vi "LVAPT_Git_Item_OnPopupMenu.vi"(11 "Object":T1) -> ()   [LabVIEW 2019]
uses:
  <resource>/Framework/Providers/API/ItemRef.ctl
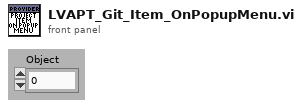
[diagram p1: front panel]
types:
  T1 = typedef "ItemRef.ctl" = u64
  T2 = enum32{"<None>", "Project", "Project / Build Specifications", "Tools", "Tools / Source Control", "Tools / Real-Time Module", "Help"}
  T3 = typedef "mxLvMenuItem.ctl" = cluster{"Menu Name":string, "Description":string, "Icon File Name":path, "Menu Tag":string, "Enabled":bool, "Checked":bool, "Separator":bool, "Batchable":bool, "Weight":i32, "Batch Mode (Ignored if Not Batchable)":enum32{"Show If All Items Support Command", "Show If Any Items Support Command"}, "Menu Location":enum32{"<None>", "Project", "Project / Build Specifications", "Tools", "Tools / Source Control", "Tools / Real-Time Module", "Help"}, "Exclude From Getting Started Window Menu":bool}
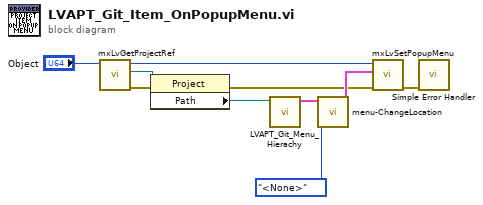
[diagram p0: block diagram]
diagram:
  n1 = call <resource>:"mxLvGetProjectRef.vi"("Item"="Object") -> ("error out"=w6:errorcluster, "Project Refnum"=w5:refnum<vi>, "Item"=w4:T1)  [unwired: 8 in]
  n2 = property class="Project"(reference=w5, error in=w6) -> (error out=w1:errorcluster, "Path"=w2:path)  [unwired: 1 out]
  n3 = call "LVAPT_Git_Menu_Hierachy.vi"("ProjectPath"=w2) -> ("Array"=w3:T3[])  [unwired: 10 in]
  n4 = call "menu-ChangeLocation.vi"("Menu Location"=T2."<None>", "Array in"=w3) -> ("Array out"=w7:T3[])  [unwired: 9 in]
  n5 = call <resource>:"mxLvSetPopupMenu.vi"("error in"=w1, "Popup Menu Items"=w7, "Item"=w4) -> ("error out"=w10:errorcluster)  [unwired: 7 in, 1 out]
  n6 = call <vilib>:"Simple Error Handler.vi"("error in (no error)"=w10) -> ()  [unwired: 4 in, 5 out]
